vi "log_message.vi"(6 "timestamp":timestamp, 7 "context":string, 8 "error in (no error)":errorcluster, 9 "level":T1=400 items=["OFF"=0, "FATAL"=100, "ERROR"=200, "WARN"=300, "INFO"=400, "DEBUG"=500, "TRACE"=600, "ALL"=65535], 10 "message":string, 11 "Queue Log Provider in":refnum<class "Queue Log Provider.lvclass">) -> (0 "error out":errorcluster, 3 "Queue Log Provider out":refnum<class "Queue Log Provider.lvclass">)   [LabVIEW 2019, in "LVCOOOP.lvlib" / "Support API.lvlib" / "Queue Log Provider.lvclass"]
uses:
  Queue Log Provider.lvclass
  Log Service/public/level.ctl
  Log Service/Log Service.lvclass
  log_message.ctl
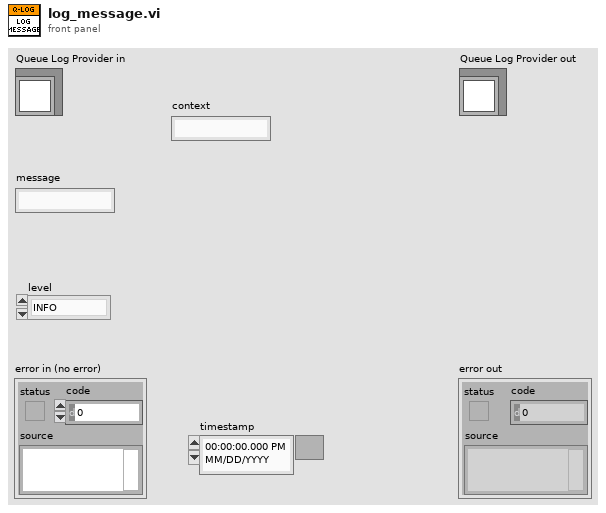
[diagram p1: front panel]
types:
  T1 = typedef "LVCOOOP.lvlib/Support API.lvlib/Log Service.lvclass/level.ctl" = u16
  T2 = typedef "LVCOOOP.lvlib/Support API.lvlib/Queue Log Provider.lvclass/log_message.ctl" = cluster{"Time Stamp":timestamp, "level":T1, "context":string, "message":string}
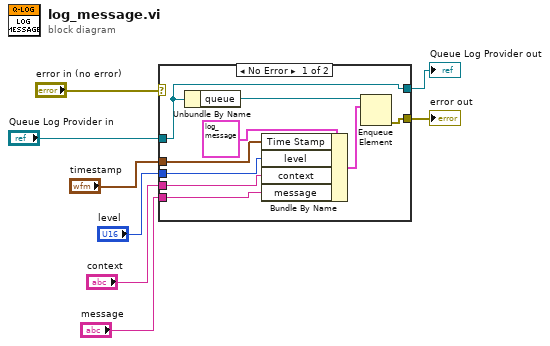
[diagram p0: block diagram]
diagram:
  n1 = case shown="No Error" "error in (no error)" {
    selector: "error in (no error)" -> [_ w19]
    tunnel: [w16 w19] -> w8
    tunnel: "timestamp" -> [w14 _]
    tunnel: "level" -> [w13 _]
    tunnel: "context" -> [w12 _]
    tunnel: "message" -> [w11 _]
    tunnel: [w9 w18] -> w2
    tunnel: "Queue Log Provider in" -> [w9 w18]
    frame No Error {
      n2 = Unbundle By Name(w9) -> ("queue"=w17:refnum<queue>)
      n3 = Bundle By Name(cluster=T2 {"Time Stamp"=timestamp(0 s since 1904-01-01), "level"=0, "context"="", "message"=""} ("element"), "Time Stamp"=w14, "level"=w13, "context"=w12, "message"=w11) -> (w10:T2)
      n4 = Enqueue Element(queue=w17, element=w10) -> (error out=w16:errorcluster)  [unwired: 2 in, 2 out]
    }
    frame Error {
    }
  }
  "error out" <- w8
  "Queue Log Provider out" <- w2
